vi "SQL_users_delete.vi"(11 "用户名":string) -> (3 "error out":errorcluster)   [LabVIEW 2014]
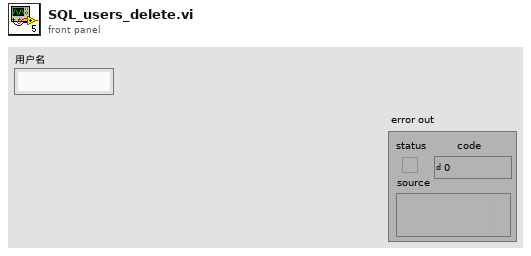
[diagram p1: front panel]
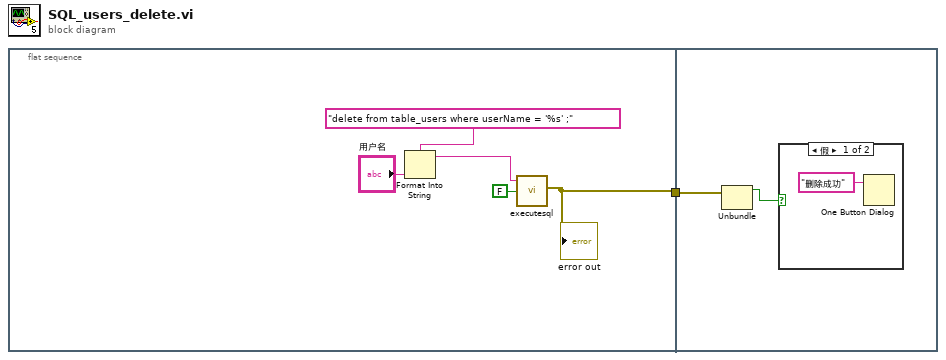
[diagram p0: block diagram]
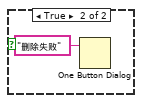
[diagram p2: hidden frame]
diagram:
  n1 = flat-sequence {
    tunnel: [w2] -> w1
    tunnel: w1 -> [w8]
    frame #0 {
      n2 = Format Into String(format string="delete from table_users where userName = '%s' ;" ("Command Text"), "用户名") -> (resulting string=w3:string)  [unwired: 2 in, 1 out]
      n3 = call "executesql.vi"("Return Data (T)"=FALSE, "Command Text"=w3) -> ("error out"=w2:errorcluster)  [unwired: 5 in, 1 out]
      "error out" <- w2
    }
    frame #1 {
      n4 = Unbundle(w8) -> ("status"=w7:bool)  [unwired: 2 out]
      n5 = case shown="假" w7 {
        frame False {
          n6 = One Button Dialog(message="删除成功" ("消息")) -> ()  [unwired: 1 in, 1 out]
        }
        frame True {
          n7 = One Button Dialog(message="删除失败" ("消息")) -> ()  [unwired: 1 in, 1 out]
        }
      }
    }
  }
